vi "Cleanup Expression.vi"(8 "error in (no error)":errorcluster, 11 "Expression Data":T1) -> (0 "error out":errorcluster)   [LabVIEW 2024, in "Output Sequencer.lvlib" / "Output Sequencer.lvclass"]
uses:
  Output Sequencer.lvclass
  Types/Expression Data.ctl
  <vilib>/LAVA/muParser/mupExpr/mupExpr.lvclass
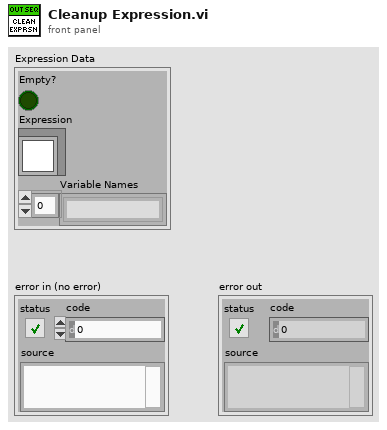
[diagram p1: front panel]
types:
  T1 = typedef "Output Sequencer.lvlib/Output Sequencer.lvclass/Expression Data.ctl" = cluster{"Empty?":bool, "Expression":refnum<class "mupExpr.lvclass">, "Variable Names":string[]}
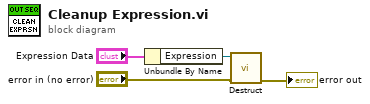
[diagram p0: block diagram]
diagram:
  n1 = Unbundle By Name("Expression Data") -> ("Expression"=w2:refnum<class "mupExpr.lvclass">)
  n2 = call-dynamic "Destruct.vi"("error in (no error)"="error in (no error)", "muExpr in"=w2) -> ("error out"=→"error out":errorcluster)  [unwired: 9 in]
